vi "valves_defcmds_C345.vi"(0 "Input solution":dbl=1.0, 1 "Add to C":dbl, 2 "Rings to open":u32, 3 "error in":errorcluster, 4 "COM4 in":refnum<k24>) -> (5 "COM4 out":refnum<k24>, 6 "Commands out":T1, 7 "error out":errorcluster)   [LabVIEW 2018]
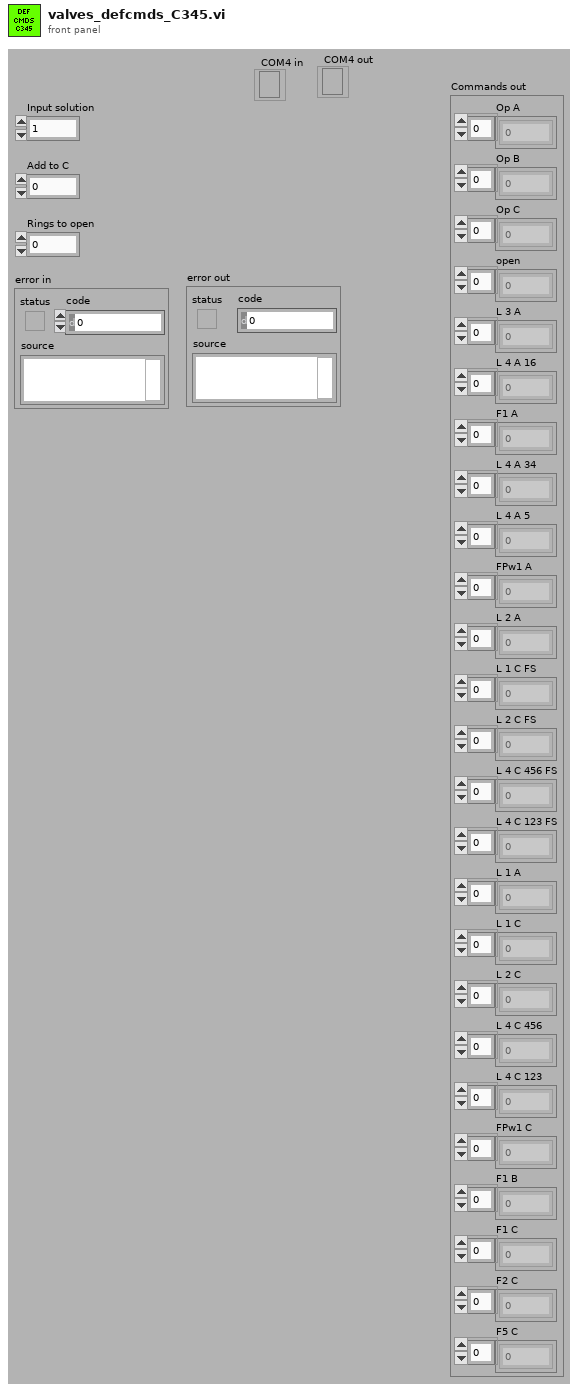
[diagram p1: front panel]
types:
  T1 = cluster{"Op A":u8[], "Op B":u8[], "Op C":u8[], "open":u8[], "L 3 A":u8[], "L 4 A 16":u8[], "F1 A":u8[], "L 4 A 34":u8[], "L 4 A 5":u8[], "FPw1 A":u8[], "L 2 A":u8[], "L 1 C FS":u8[], "L 2 C FS":u8[], "L 4 C 456 FS":u8[], "L 4 C 123 FS":u8[], "L 1 A":u8[], "L 1 C":u8[], "L 2 C":u8[], "L 4 C 456":u8[], "L 4 C 123":u8[], "FPw1 C":u8[], "F1 B":u8[], "F1 C":u8[], "F2 C":u8[], "F5 C":u8[]}
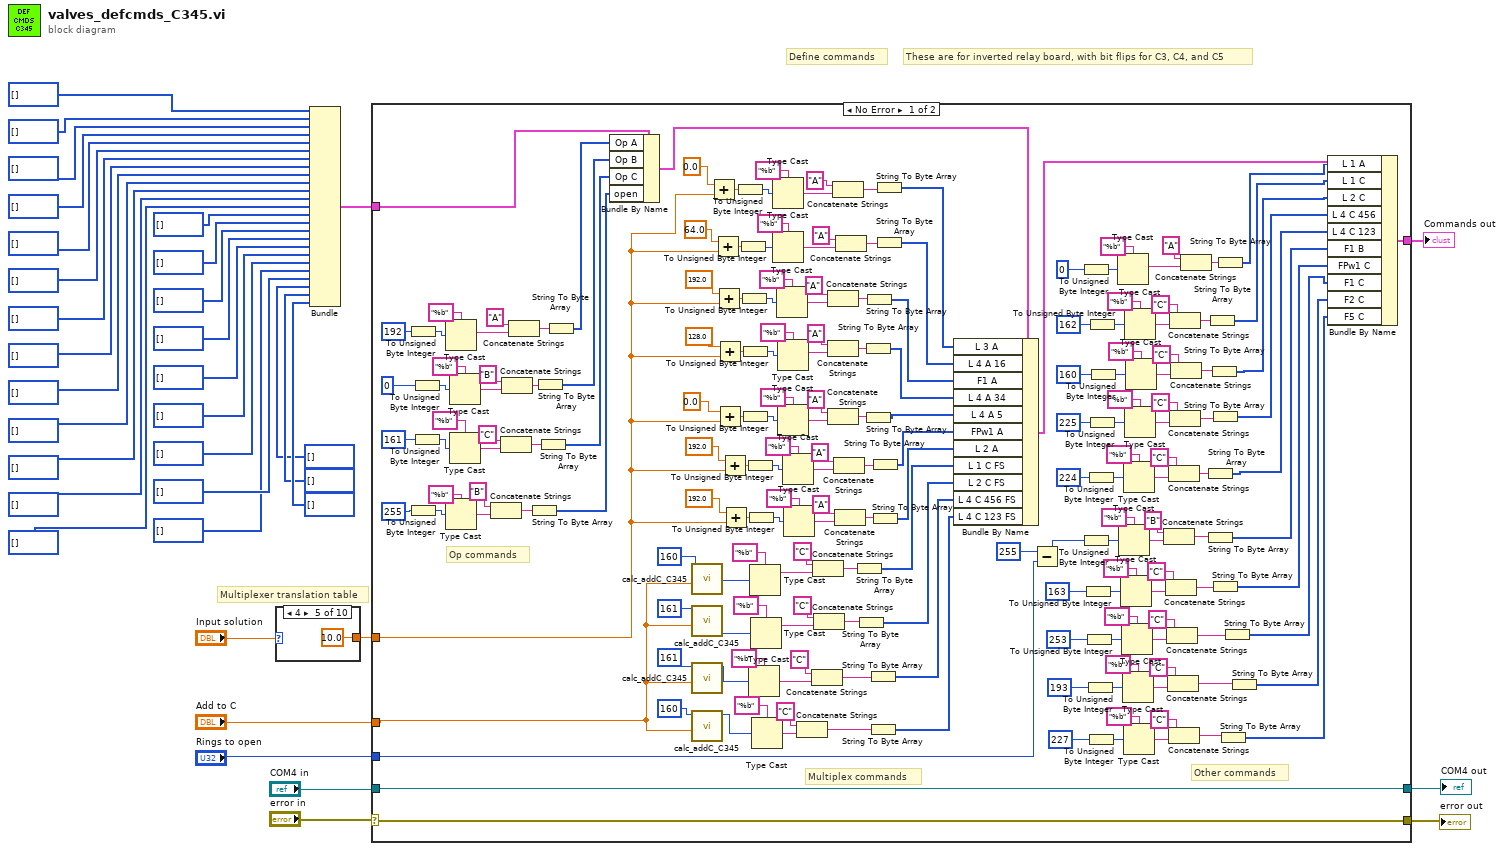
[diagram p0: block diagram]
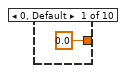
[diagram p3: hidden frame]
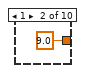
[diagram p4: hidden frame]
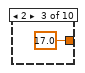
[diagram p5: hidden frame]
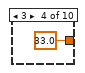
[diagram p6: hidden frame]
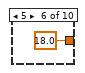
[diagram p7: hidden frame]
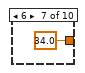
[diagram p8: hidden frame]
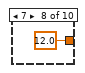
[diagram p9: hidden frame]
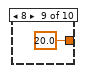
[diagram p10: hidden frame]
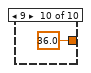
[diagram p11: hidden frame]
diagram:
  # "These are for inverted relay board, with bit flips for C3, C4, and C5"
  # "Define commands"
  # "Multiplexer translation table"
  n1 = case shown="4" "Input solution" {
    tunnel: [0.0 ("open flush") 9.0 ("open flush") 17.0 ("open flush") 33.0 ("open flush") 10.0 ("open flush") 18.0 ("open flush") 34.0 ("open flush") 12.0 ("open flush") 20.0 ("open flush") 36.0 ("open flush")] -> w31
    frame 0, Default {
    }
    frame 1 {
    }
    frame 2 {
    }
    frame 3 {
    }
    frame 4 {
    }
    frame 5 {
    }
    frame 6 {
    }
    frame 7 {
    }
    frame 8 {
    }
    frame 9 {
    }
  }
  n2 = Bundle("Op A"=u8[] [], "Op B"=u8[] [], "Op C"=u8[] [], "open"=u8[] [], "L 3 A"=u8[] [], "L 4 A 16"=u8[] [], "F1 A"=u8[] [], "L 4 A 34"=u8[] [], "L 4 A 5"=u8[] [], "FPw1 A"=u8[] [], "L 2 A"=u8[] [], "L 1 C FS"=u8[] [], "L 2 C FS"=u8[] [], "L 4 C 456 FS"=u8[] [], "L 4 C 123 FS"=u8[] [], "L 1 A"=u8[] [], "L 1 C"=u8[] [], "L 2 C"=u8[] [], "L 4 C 456"=u8[] [], "L 4 C 123"=u8[] [], "FPw1 C"=u8[] [], "F1 B"=u8[] [], "F1 C"=u8[] [], "F2 C"=u8[] [], "F5 C"=u8[] []) -> (w2:T1)  [unwired: 1 in]
  n3 = case shown="No Error" "error in" {
    selector: "error in" -> [w113 w239]
    tunnel: w31 -> [w53 _]
    tunnel: "Add to C" -> [w49 _]
    tunnel: "Rings to open" -> [w57 _]
    tunnel: [w113 w239] -> w35
    tunnel: "COM4 in" -> [w112 w240]
    tunnel: [w112 w240] -> w28
    tunnel: w2 -> [w110 w238]
    tunnel: [w59 w238] -> w1
    frame No Error {
      # "Other commands"
      # "Multiplex commands"
      # "Op commands"
      n4 = To Unsigned Byte Integer(number=u8 192) -> (unsigned 8bit integer=w223:u8)
      n5 = To Unsigned Byte Integer(number=u8 255) -> (unsigned 8bit integer=w222:u8)
      n6 = To Unsigned Byte Integer(number=u8 0) -> (unsigned 8bit integer=w226:u8)
      n7 = To Unsigned Byte Integer(number=u8 161) -> (unsigned 8bit integer=w231:u8)
      n8 = Type Cast(type="%b", x=w223) -> (*(type *) &x=w224:string)
      n9 = Type Cast(type="%b", x=w222) -> (*(type *) &x=w221:string)
      n10 = Type Cast(type="%b", x=w226) -> (*(type *) &x=w227:string)
      n11 = Type Cast(type="%b", x=w231) -> (*(type *) &x=w232:string)
      n12 = Concatenate Strings("B", w221) -> (w107:string)
      n13 = Concatenate Strings("C", w232) -> (w105:string)
      n14 = Concatenate Strings("B", w227) -> (w103:string)
      n15 = Concatenate Strings("A", w224) -> (w109:string)
      n16 = String To Byte Array(string=w107) -> (unsigned byte array=w106:u8[])
      n17 = String To Byte Array(string=w103) -> (unsigned byte array=w102:u8[])
      n18 = String To Byte Array(string=w105) -> (unsigned byte array=w104:u8[])
      n19 = String To Byte Array(string=w109) -> (unsigned byte array=w108:u8[])
      n20 = Bundle By Name(cluster=w110, "Op A"=w108, "Op B"=w102, "Op C"=w104, "open"=w106) -> (w115:T1)
      n21 = call "calc_addC_C345.vi"("Add to C"=w49, "Input U8"=u8 160 ("number")) -> ("Output U8"=w55:u8)  [unwired: 9 in]
      n22 = call "calc_addC_C345.vi"("Add to C"=w49, "Input U8"=u8 161 ("number")) -> ("Output U8"=w46:u8)  [unwired: 9 in]
      n23 = call "calc_addC_C345.vi"("Add to C"=w49, "Input U8"=u8 161 ("number")) -> ("Output U8"=w47:u8)  [unwired: 9 in]
      n24 = call "calc_addC_C345.vi"("Add to C"=w49, "Input U8"=u8 160 ("number")) -> ("Output U8"=w48:u8)  [unwired: 9 in]
      n25 = Add(x=0.0, y=w53) -> (x+y=w192:dbl)
      n26 = Add(x=64.0, y=w53) -> (x+y=w198:dbl)
      n27 = Add(x=192.0, y=w53) -> (x+y=w203:dbl)
      n28 = Add(x=128.0, y=w53) -> (x+y=w210:dbl)
      n29 = Add(x=0.0, y=w53) -> (x+y=w215:dbl)
      n30 = Add(x=192.0, y=w53) -> (x+y=w185:dbl)
      n31 = Add(x=192.0, y=w53) -> (x+y=w167:dbl)
      n32 = To Unsigned Byte Integer(number=w192) -> (unsigned 8bit integer=w188:u8)
      n33 = To Unsigned Byte Integer(number=w198) -> (unsigned 8bit integer=w194:u8)
      n34 = To Unsigned Byte Integer(number=w203) -> (unsigned 8bit integer=w200:u8)
      n35 = To Unsigned Byte Integer(number=w210) -> (unsigned 8bit integer=w206:u8)
      n36 = To Unsigned Byte Integer(number=w215) -> (unsigned 8bit integer=w211:u8)
      n37 = To Unsigned Byte Integer(number=w185) -> (unsigned 8bit integer=w182:u8)
      n38 = To Unsigned Byte Integer(number=w167) -> (unsigned 8bit integer=w164:u8)
      n39 = Type Cast(type="%b", x=w47) -> (*(type *) &x=w176:string)
      n40 = Type Cast(type="%b", x=w55) -> (*(type *) &x=w170:string)
      n41 = Type Cast(type="%b", x=w46) -> (*(type *) &x=w173:string)
      n42 = Type Cast(type="%b", x=w48) -> (*(type *) &x=w179:string)
      n43 = Type Cast(type="%b", x=w188) -> (*(type *) &x=w189:string)
      n44 = Type Cast(type="%b", x=w194) -> (*(type *) &x=w195:string)
      n45 = Type Cast(type="%b", x=w200) -> (*(type *) &x=w201:string)
      n46 = Type Cast(type="%b", x=w206) -> (*(type *) &x=w207:string)
      n47 = Type Cast(type="%b", x=w211) -> (*(type *) &x=w212:string)
      n48 = Type Cast(type="%b", x=w182) -> (*(type *) &x=w183:string)
      n49 = Type Cast(type="%b", x=w164) -> (*(type *) &x=w165:string)
      n50 = Concatenate Strings("C", w179) -> (w81:string)
      n51 = Concatenate Strings("C", w176) -> (w83:string)
      n52 = Concatenate Strings("C", w170) -> (w87:string)
      n53 = Concatenate Strings("C", w173) -> (w85:string)
      n54 = Concatenate Strings("A", w201) -> (w97:string)
      n55 = Concatenate Strings("A", w207) -> (w95:string)
      n56 = Concatenate Strings("A", w212) -> (w93:string)
      n57 = Concatenate Strings("A", w189) -> (w101:string)
      n58 = Concatenate Strings("A", w183) -> (w91:string)
      n59 = Concatenate Strings("A", w165) -> (w89:string)
      n60 = Concatenate Strings("A", w195) -> (w99:string)
      n61 = String To Byte Array(string=w87) -> (unsigned byte array=w86:u8[])
      n62 = String To Byte Array(string=w85) -> (unsigned byte array=w84:u8[])
      n63 = String To Byte Array(string=w95) -> (unsigned byte array=w94:u8[])
      n64 = String To Byte Array(string=w93) -> (unsigned byte array=w92:u8[])
      n65 = String To Byte Array(string=w97) -> (unsigned byte array=w96:u8[])
      n66 = String To Byte Array(string=w83) -> (unsigned byte array=w82:u8[])
      n67 = String To Byte Array(string=w81) -> (unsigned byte array=w80:u8[])
      n68 = String To Byte Array(string=w91) -> (unsigned byte array=w90:u8[])
      n69 = String To Byte Array(string=w89) -> (unsigned byte array=w88:u8[])
      n70 = String To Byte Array(string=w101) -> (unsigned byte array=w100:u8[])
      n71 = String To Byte Array(string=w99) -> (unsigned byte array=w98:u8[])
      n72 = Bundle By Name(cluster=w115, "L 3 A"=w100, "L 4 A 16"=w98, "F1 A"=w96, "L 4 A 34"=w94, "L 4 A 5"=w92, "FPw1 A"=w90, "L 2 A"=w88, "L 1 C FS"=w86, "L 2 C FS"=w84, "L 4 C 456 FS"=w82, "L 4 C 123 FS"=w80) -> (w114:T1)
      n73 = Subtract(x=u32 255, y=w57) -> (x-y=w56:u32)
      n74 = To Unsigned Byte Integer(number=u8 0) -> (unsigned 8bit integer=w155:u8)
      n75 = To Unsigned Byte Integer(number=w56) -> (unsigned 8bit integer=w160:u8)
      n76 = To Unsigned Byte Integer(number=u8 163) -> (unsigned 8bit integer=w153:u8)
      n77 = To Unsigned Byte Integer(number=u8 253) -> (unsigned 8bit integer=w148:u8)
      n78 = To Unsigned Byte Integer(number=u8 193) -> (unsigned 8bit integer=w143:u8)
      n79 = To Unsigned Byte Integer(number=u8 224) -> (unsigned 8bit integer=w118:u8)
      n80 = To Unsigned Byte Integer(number=u8 227) -> (unsigned 8bit integer=w139:u8)
      n81 = To Unsigned Byte Integer(number=u8 162) -> (unsigned 8bit integer=w133:u8)
      n82 = To Unsigned Byte Integer(number=u8 225) -> (unsigned 8bit integer=w124:u8)
      n83 = To Unsigned Byte Integer(number=u8 160) -> (unsigned 8bit integer=w128:u8)
      n84 = Type Cast(type="%b", x=w155) -> (*(type *) &x=w156:string)
      n85 = Type Cast(type="%b", x=w160) -> (*(type *) &x=w161:string)
      n86 = Type Cast(type="%b", x=w153) -> (*(type *) &x=w154:string)
      n87 = Type Cast(type="%b", x=w148) -> (*(type *) &x=w149:string)
      n88 = Type Cast(type="%b", x=w143) -> (*(type *) &x=w144:string)
      n89 = Type Cast(type="%b", x=w118) -> (*(type *) &x=w119:string)
      n90 = Type Cast(type="%b", x=w139) -> (*(type *) &x=w140:string)
      n91 = Type Cast(type="%b", x=w133) -> (*(type *) &x=w134:string)
      n92 = Type Cast(type="%b", x=w124) -> (*(type *) &x=w125:string)
      n93 = Type Cast(type="%b", x=w128) -> (*(type *) &x=w129:string)
      n94 = Concatenate Strings("B", w161) -> (w69:string)
      n95 = Concatenate Strings("C", w154) -> (w67:string)
      n96 = Concatenate Strings("C", w149) -> (w65:string)
      n97 = Concatenate Strings("C", w144) -> (w63:string)
      n98 = Concatenate Strings("C", w119) -> (w71:string)
      n99 = Concatenate Strings("C", w140) -> (w61:string)
      n100 = Concatenate Strings("C", w134) -> (w77:string)
      n101 = Concatenate Strings("C", w125) -> (w73:string)
      n102 = Concatenate Strings("C", w129) -> (w75:string)
      n103 = Concatenate Strings("A", w156) -> (w79:string)
      n104 = String To Byte Array(string=w71) -> (unsigned byte array=w70:u8[])
      n105 = String To Byte Array(string=w69) -> (unsigned byte array=w68:u8[])
      n106 = String To Byte Array(string=w77) -> (unsigned byte array=w76:u8[])
      n107 = String To Byte Array(string=w75) -> (unsigned byte array=w74:u8[])
      n108 = String To Byte Array(string=w73) -> (unsigned byte array=w72:u8[])
      n109 = String To Byte Array(string=w67) -> (unsigned byte array=w66:u8[])
      n110 = String To Byte Array(string=w79) -> (unsigned byte array=w78:u8[])
      n111 = String To Byte Array(string=w61) -> (unsigned byte array=w60:u8[])
      n112 = String To Byte Array(string=w65) -> (unsigned byte array=w64:u8[])
      n113 = String To Byte Array(string=w63) -> (unsigned byte array=w62:u8[])
      n114 = Bundle By Name(cluster=w114, "L 1 A"=w78, "L 1 C"=w76, "L 2 C"=w74, "L 4 C 456"=w72, "L 4 C 123"=w70, "F1 B"=w68, "FPw1 C"=w66, "F1 C"=w64, "F2 C"=w62, "F5 C"=w60) -> (w59:T1)
    }
    frame Error {
    }
  }
  "error out" <- w35
  "COM4 out" <- w28
  "Commands out" <- w1
